vi "Get Thing Details.vi"(8 "error in (no error)":errorcluster, 10 "Name":string, 11 "IoT Session in":refnum<class "IoT Session.lvclass">) -> (0 "error out":errorcluster, 2 "Thing":T1, 3 "IoT Session out":refnum<class "IoT Session.lvclass">)   [LabVIEW 2015, in "NI_AWS_IoT.lvlib" / "IoT Session.lvclass"]
uses:
  IoT Session.lvclass
  Thing.ctl
  Core/HTTP Request/Name Value Pair.ctl
  Core/HTTP Request/Request Options.ctl
  Core/HTTP Request/Region handling.ctl
  Core/HTTP Request/URL formatting.ctl
  Core/HTTP Request/HTTP Request.lvclass
  NI_AWS_IoT.lvlib
  JSON Parsing/NI_JSON Parsing.lvlib
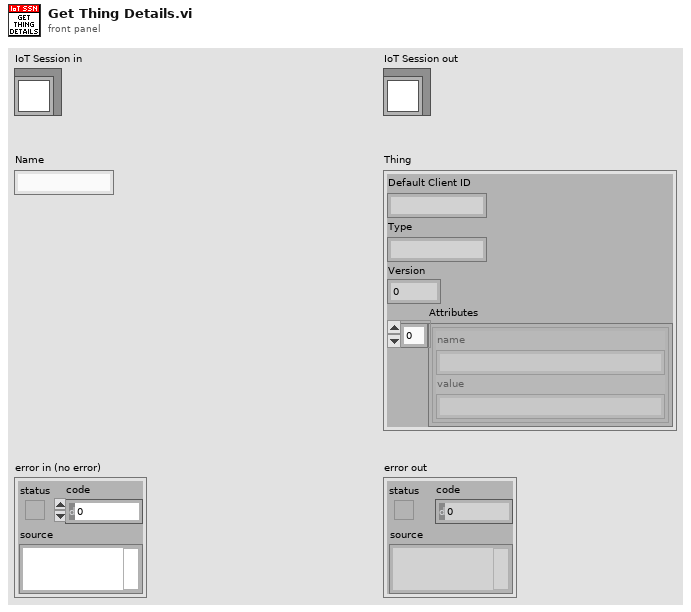
[diagram p1: front panel]
types:
  T1 = typedef "NI_AWS_IoT.lvlib/Thing.ctl" = cluster{"Default Client ID":string, "Type":string, "Version":i32, "Attributes":T2[]}
  T2 = typedef "NI_AWS_Core.lvlib/HTTP Request.lvclass/Name Value Pair.ctl" = cluster{"name":string, "value":string}
  T3 = typedef "NI_AWS_Core.lvlib/HTTP Request.lvclass/Request Options.ctl" = cluster{"request headers":T2[], "request parameters":T2[], "request body":string, "region handling":T4, "URL formatting":T5}
  T4 = typedef "NI_AWS_Core.lvlib/HTTP Request.lvclass/Region handling.ctl" = enum16{"use region everywhere", "use region (authentication only)", "use region (URL only)", "ignore region everwhere"}
  T5 = typedef "NI_AWS_Core.lvlib/HTTP Request.lvclass/URL formatting.ctl" = enum16{"region-", "region."}
  T6 = typedef "NI_AWS_Core.lvlib/HTTP Request.lvclass/Response.ctl" = cluster{"Headers":string, "Body":string}
  T7 = typedef "NI_JSON Parsing.lvlib/Name Value Pair.ctl" = cluster{"name":string, "value":string}
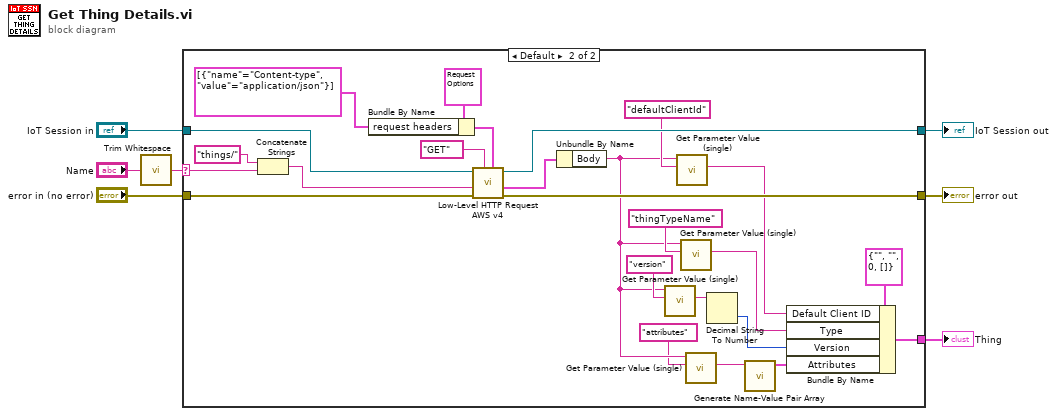
[diagram p0: block diagram]
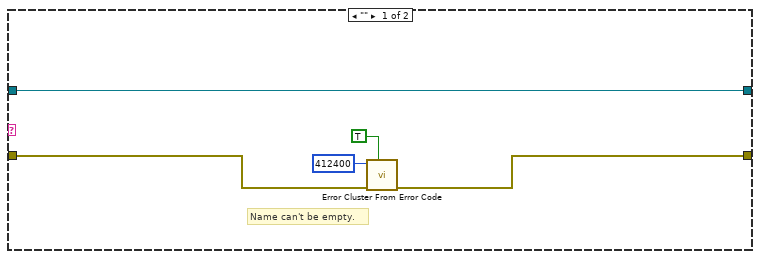
[diagram p2: hidden frame]
diagram:
  n1 = call <vilib>:"Trim Whitespace.vi"("string"="Name") -> ("trimmed string"=w1:string)  [unwired: 1 in]
  n2 = case shown="Default" w1 {
    selector: w1 -> [_ w13]
    tunnel: "error in (no error)" -> [w10 w37]
    tunnel: [w9 w36] -> w6
    tunnel: [w8 w35] -> w5
    tunnel: "IoT Session in" -> [w8 w34]
    tunnel: [_ w25] -> w2
    frame "" {
      # "Name can't be empty."
      n3 = call <vilib>:"Error Cluster From Error Code.vi"("show call chain? (False)"=TRUE, "error in (no error)"=w10, "error code (0)"=412400) -> ("error out"=w9:errorcluster)  [unwired: 6 in]
    }
    frame Default {
      n4 = Concatenate Strings("things/" ("string"), w13) -> (w30:string)
      n5 = Bundle By Name(cluster=T3 {"request headers"=[], "request parameters"=[], "request body"="", "region handling"=enum."use region everywhere", "URL formatting"=enum."region."} ("Request Options"), "request headers"=T2[] [{"name"="Content-type", "value"="application/json"}]) -> (w32:T3)
      n6 = call "Low-Level HTTP Request AWS v4.vi"("Request Options"=w32, "HTTP-Verb"="GET", "error in (no error)"=w37, "URL Suffix"=w30, "AWS Core in"=w34) -> ("error out"=w36:errorcluster, "Response"=w27:T6, "AWS Core out"=w35:refnum<class "IoT Session.lvclass">)  [unwired: 3 in, 1 out]
      n7 = Unbundle By Name(w27) -> ("Body"=w17:string)
      n8 = call "Get Parameter Value (single).vi"("Parameter Name"="version", "JSON"=w17) -> ("Parameter Value"=w19:string)  [unwired: 6 in, 3 out]
      n9 = call "Get Parameter Value (single).vi"("Parameter Name"="defaultClientId", "JSON"=w17) -> ("Parameter Value"=w23:string)  [unwired: 6 in, 3 out]
      n10 = call "Get Parameter Value (single).vi"("Parameter Name"="thingTypeName", "JSON"=w17) -> ("Parameter Value"=w21:string)  [unwired: 6 in, 3 out]
      n11 = call "Get Parameter Value (single).vi"("Parameter Name"="attributes", "JSON"=w17) -> ("Parameter Value"=w15:string)  [unwired: 6 in, 3 out]
      n12 = Decimal String To Number(string=w19) -> (number=w18:i32)  [unwired: 2 in, 1 out]
      n13 = call "Generate Name-Value Pair Array.vi"("Name-Value Pair JSON"=w15) -> ("Name-Value Pairs"=w14:T7[])  [unwired: 10 in]
      n14 = Bundle By Name(cluster=T1 {"Default Client ID"="", "Type"="", "Version"=0, "Attributes"=[]} ("Thing"), "Default Client ID"=w23, "Type"=w21, "Version"=w18, "Attributes"=w14) -> (w25:T1)
    }
  }
  "error out" <- w6
  "IoT Session out" <- w5
  "Thing" <- w2
